vi "Get ID.vi"(8 "error in (no error)":errorcluster, 11 "2DPanelBlank in":refnum<class "2DPanelBlank.lvclass">) -> (0 "error out":errorcluster, 2 "ID":i32 format="%08x", 3 "2DPanelBlank out":refnum<class "2DPanelBlank.lvclass">)   [LabVIEW 2020, in "OOPanel.lvlib" / "2DPanelBlank.lvclass"]
uses:
  2DPanelBlank.lvclass
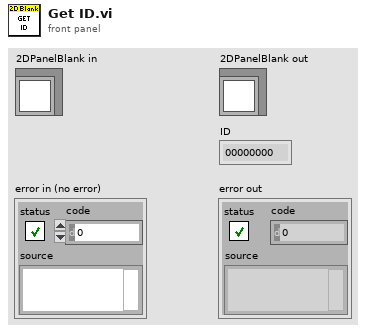
[diagram p1: front panel]
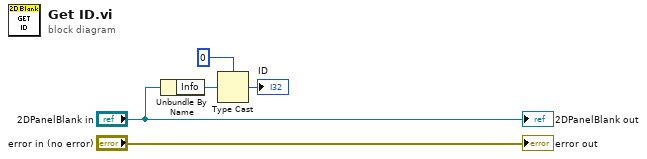
[diagram p0: block diagram]
diagram:
  n1 = Unbundle By Name("2DPanelBlank in") -> ("Info"=w3:refnum<data-value>)
  n2 = Type Cast(type=0, x=w3) -> (*(type *) &x=→"ID":i32)
  "error out" <- "error in (no error)"
  "2DPanelBlank out" <- "2DPanelBlank in"
